vi "CB Holonomic Drivebase Double Model.vi"() -> ()   [LabVIEW 2020]
uses:
  CB State Space.ctl
  <vilib>/Analysis/Matrix/Datatypes/RealMatrix.ctl
  <vilib>/Analysis/Matrix/Numeric/Conversions/Array To Matrix - RA2.vi
  <vilib>/Analysis/Matrix/NI_Matrix.lvlib
panel:
  out "State Space Model":T1
  in  "dt":dbl=-1.0
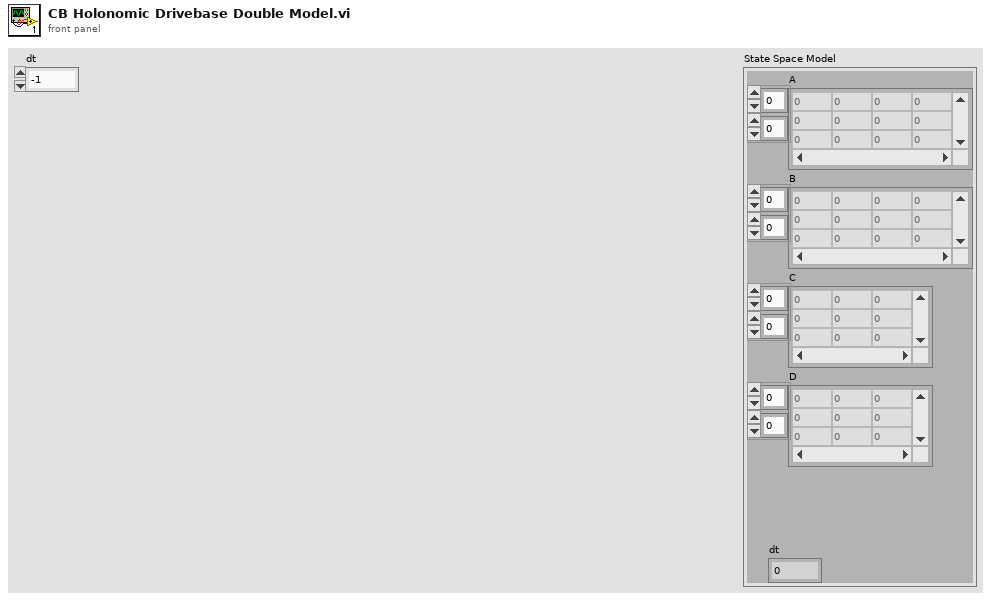
[diagram p1: front panel]
types:
  T1 = typedef "CB State Space.ctl" = cluster{"A":T2, "B":T2, "C":T2, "D":T2, "dt":dbl}
  T2 = typedef "NI_Matrix.lvlib/RealMatrix.ctl" = dbl[][]
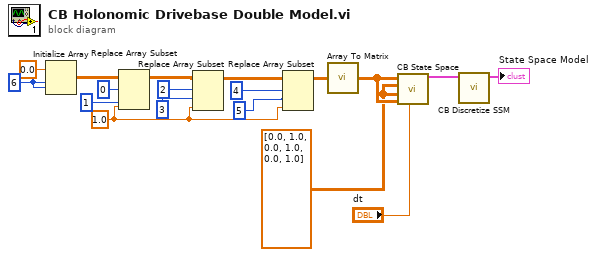
[diagram p0: block diagram]
diagram:
  w1 = T2 [[0.0], [1.0], [0.0], [1.0], [0.0], [1.0]] ("B")
  w7 = 1.0 ("new element/subarray")
  w18 = 6 ("dimension size")
  n1 = Initialize Array(0.0 ("element"), w18, w18) -> (w16:dbl[][])
  n2 = Replace Array Subset(array=w16, new element=w7, index (row)=0, index (col)=1 ("disabled index (col)")) -> (w13:dbl[][])
  n3 = Replace Array Subset(array=w13, new element=w7, index (row)=2, index (col)=3 ("disabled index (col)")) -> (w10:dbl[][])
  n4 = Replace Array Subset(array=w10, new element=w7, index (row)=4, index (col)=5 ("index (row)")) -> (w6:dbl[][])
  n5 = call-poly <vilib>:"Array To Matrix.vi"("Real 2D Array"=w6) -> ("Real Matrix"=w2:T2)
  n6 = call "CB State Space.vi"("dt"="dt", "D"=w2, "C"=w1, "B"=w1, "A"=w2) -> ("State Space Model"=w4:T1)  [unwired: 5 in, 1 out]
  n7 = call "CB Discretize SSM.vi"("Cont SSM"=w4) -> ("State Space Model"=→"State Space Model":T1)  [unwired: 10 in]
